vi "Timer.vi"(10 "Action":enum16{"Reset", "Get"}(ring)=enum."Get") -> (2 "Elapsed":bool)   [LabVIEW 2023]
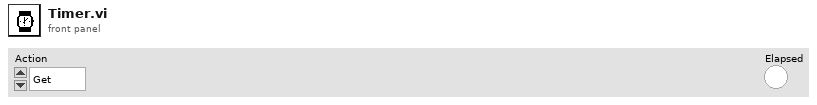
[diagram p1: front panel]
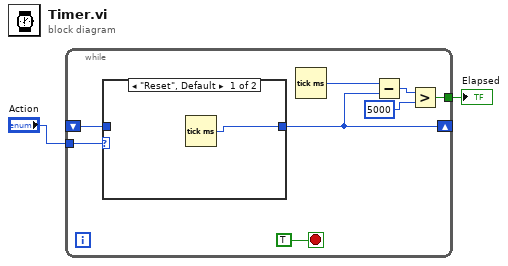
[diagram p0: block diagram]
diagram:
  n1 = while {
    shift-right: [w6] -> _
    shift-left: _ -> [w8]
    tunnel: "Action" -> [w9]
    tunnel: [w3] -> w1
    stop <- TRUE stop-if-true
    n2 = case shown="\"Reset\", Default" w9 {
      tunnel: [w11 w12] -> w6
      tunnel: w8 -> [_ w12]
      frame "Reset", Default {
        n3 = Tick Count (ms)() -> (millisecond timer value=w11:u32)
      }
      frame "Get" {
      }
    }
    n4 = Tick Count (ms)() -> (millisecond timer value=w7:u32)
    n5 = Subtract(x=w7, y=w6) -> (x-y=w5:u32)
    n6 = Greater?(x=w5, y=u32 5000) -> (0:w3:bool)
  }
  "Elapsed" <- w1
